vi "Write object configuration.vi"(6 "Object name":string, 8 "Error In":errorcluster, 9 "Configuration":variant, 10 "File path":path, 11 "object":refnum<class>) -> (0 "Error Out":errorcluster, 1 "Section out":string, 2 "File path out":path)   [LabVIEW 2015]
uses:
  <vilib>/Utility/config.llb/NI_LVConfig.lvlib
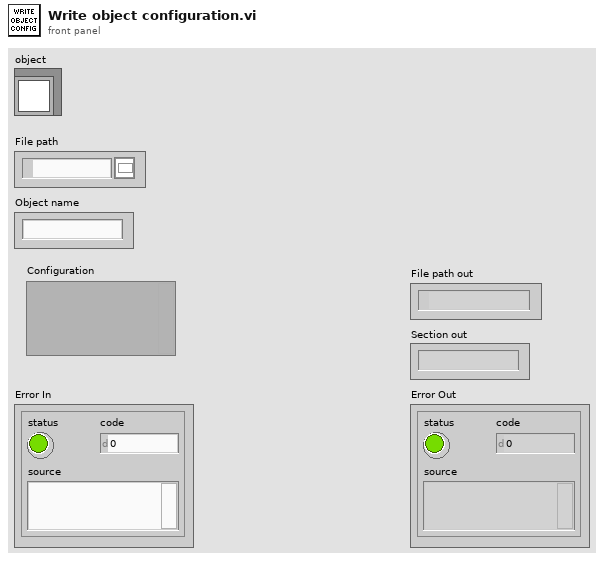
[diagram p1: front panel]
types:
  T1 = typedef "NI_LVConfig.lvlib/Config Data RefNum.ctl" = refnum<k1>
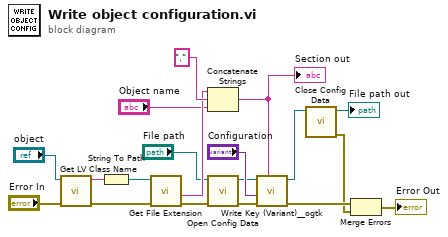
[diagram p0: block diagram]
diagram:
  n1 = call <vilib>:"Get LV Class Name.vi"("error in (no error)"="Error In", "object"="object") -> ("error out"=w16:errorcluster, "class name"=w18:string)  [unwired: 8 in]
  n2 = String To Path(string=w18) -> (path=w14:path)
  n3 = call <vilib>:"Get File Extension.vi"("error in (no error)"=w16, "file"=w14) -> ("error out"=w17:errorcluster, "filename without extension"=w15:string)  [unwired: 5 in, 3 out]
  n4 = Concatenate Strings(w15, "." ("string"), "Object name") -> (w8:string)
  "Section out" <- w8
  n5 = call <vilib>:"Open Config Data.vi"("error in (no error)"=w17, "configuration file path"="File path") -> ("error out"=w9:errorcluster, "refnum"=w10:T1)  [unwired: 7 in, 1 out]
  n6 = call <userlib>:"Write Key (Variant)__ogtk.vi"("section"=w8, "error in (no error)"=w9, "key-value"="Configuration", "refnum"=w10) -> ("error out"=w6:errorcluster, "refnum out"=w7:T1)  [unwired: 6 in]
  n7 = call <vilib>:"Close Config Data.vi"("refnum"=w7) -> ("error out"=w5:errorcluster, "file path"=→"File path out":path)  [unwired: 9 in]
  n8 = Merge Errors(w6, w5) -> (→"Error Out":errorcluster)
